vi "Copy Template.vi"(11 "error in (no error)":errorcluster) -> (15 "error out":errorcluster)   [LabVIEW 2021, in "G Plug-in Migrator.lvlib"]
uses:
  G Plug-in Migrator.lvlib
  Generator/_InstrumentStudio Plug-In Editor/controls/Data Holder.ctl
  Generator/_InstrumentStudio Plug-In Editor/InstrumentStudio Plug-In Editor.lvlib
  Migrator Reusables/Migrator Reusables.lvlib
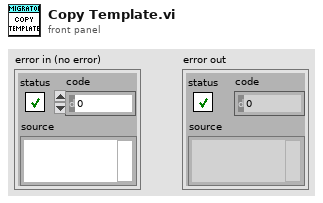
[diagram p1: front panel]
types:
  T1 = typedef "InstrumentStudio Plug-In Editor.lvlib/Data Holder.ctl" = cluster{"project ref":refnum<vi>, "Name":string, "Plugin Group Name":string}
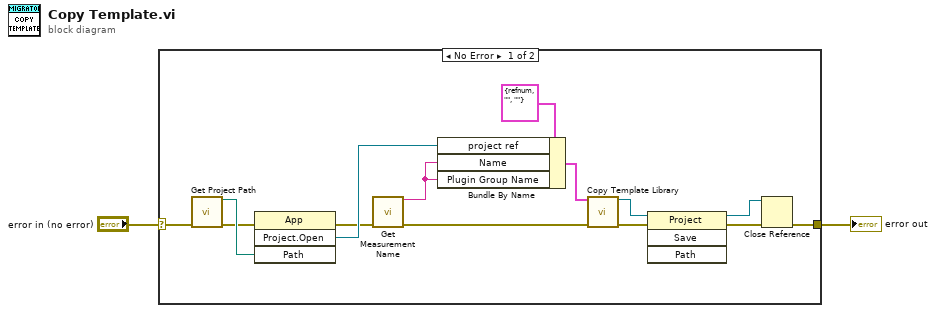
[diagram p0: block diagram]
diagram:
  n1 = case shown="No Error" "error in (no error)" {
    selector: "error in (no error)" -> [w13 w17]
    tunnel: [w5 w17] -> w2
    frame No Error {
      n2 = call "Get Project Path.vi"("error in (no error)"=w13) -> ("Project Path Out"=w15:path, "error out"=w14:errorcluster)  [unwired: 13 in]
      n3 = invoke class="App" method="Project.Open"(error in=w14, "Path"=w15) -> (error out=w9:errorcluster, "Project:Open"=w11:refnum<vi>)  [unwired: 2 in, 2 out]
      n4 = call "Get Measurement Name.vi"("error in (no error)"=w9) -> ("Name Out"=w3:string, "error out"=w10:errorcluster)  [unwired: 13 in]
      n5 = Bundle By Name(cluster=T1 {"project ref"=refnum, "Name"="", "Plugin Group Name"=""} ("Configuration"), "project ref"=w11, "Name"=w3, "Plugin Group Name"=w3) -> (w12:T1)
      n6 = call "Copy Template Library.vi"("configuration"=w12, "error in"=w10) -> ("project ref out"=w8:refnum<vi>, "error out"=w7:errorcluster)  [unwired: 12 in]
      n7 = invoke class="Project" method="Save"(reference=w8, error in=w7) -> (reference out=w4:refnum<vi>, error out=w6:errorcluster)  [unwired: 2 in, 2 out]
      n8 = Close Reference(reference=w4, error in (no error)=w6) -> (error out=w5:errorcluster)
    }
    frame Error {
    }
  }
  "error out" <- w2
